vi "Relay Command Generator.vi"(1 "Relay":u16(ring) items=["1", "2", "3", "4", "5", "6", "7", "8", "9", "10", "11", "12", "13", "14", "15", "16"], 3 "On/Off":bool=TRUE) -> (8 "Generated Command":string)   [LabVIEW 2018]
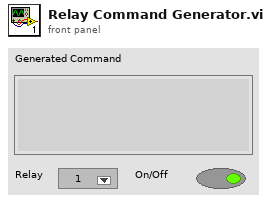
[diagram p1: front panel]
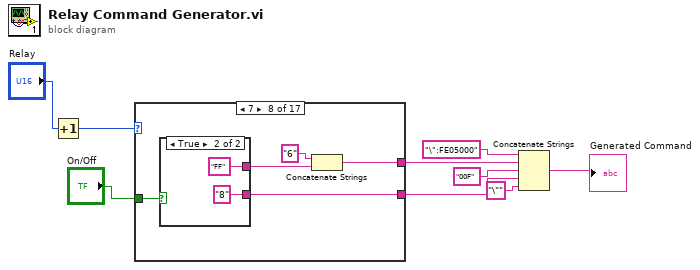
[diagram p0: block diagram]
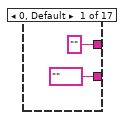
[diagram p2: hidden frame]
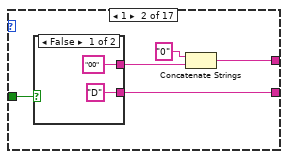
[diagram p3: hidden frame]
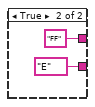
[diagram p4: hidden frame]
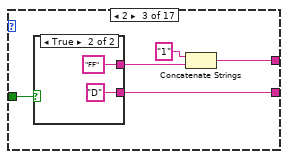
[diagram p5: hidden frame]
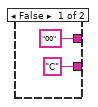
[diagram p6: hidden frame]
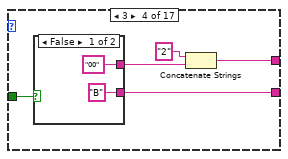
[diagram p7: hidden frame]
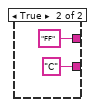
[diagram p8: hidden frame]
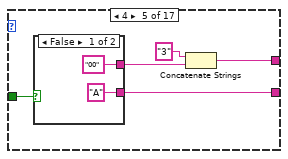
[diagram p9: hidden frame]
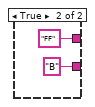
[diagram p10: hidden frame]
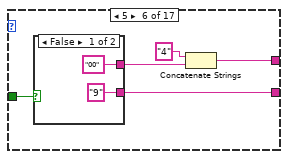
[diagram p11: hidden frame]
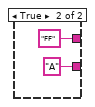
[diagram p12: hidden frame]
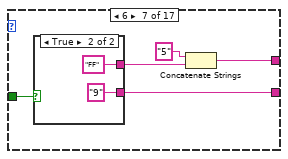
[diagram p13: hidden frame]
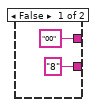
[diagram p14: hidden frame]
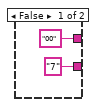
[diagram p15: hidden frame]
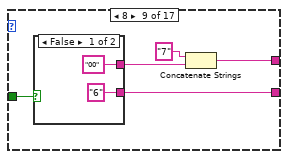
[diagram p16: hidden frame]
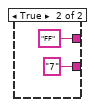
[diagram p17: hidden frame]
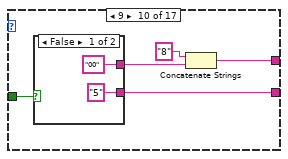
[diagram p18: hidden frame]
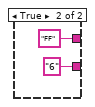
[diagram p19: hidden frame]
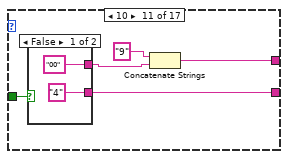
[diagram p20: hidden frame]
diagram:
  n1 = Increment(x="Relay") -> (x+1=w6:u16)
  n2 = case shown="7" w6 {
    tunnel: ["" w12 w21 w30 w39 w48 w57 w66 w75 w84 w93 w102 w111 w120 w129 w138 w147] -> w4
    tunnel: ["" w16 w25 w34 w43 w52 w61 w70 w79 w88 w97 w106 w115 w124 w133 w142 w151] -> w5
    tunnel: "On/Off" -> [_ w15 w24 w33 w42 w51 w60 w69 w78 w87 w96 w105 w114 w123 w132 w141 w150]
    frame 0, Default {
    }
    frame 1 {
      n3 = case shown="False" w15 {
        tunnel: ["00" "FF"] -> w13
        tunnel: ["D" "E"] -> w16
        frame False {
        }
        frame True {
        }
      }
      n4 = Concatenate Strings("0", w13) -> (w12:string)
    }
    frame 2 {
      n5 = case shown="True" w24 {
        tunnel: ["00" "FF"] -> w22
        tunnel: ["C" "D"] -> w25
        frame False {
        }
        frame True {
        }
      }
      n6 = Concatenate Strings("1", w22) -> (w21:string)
    }
    frame 3 {
      n7 = case shown="False" w33 {
        tunnel: ["00" "FF"] -> w31
        tunnel: ["B" "C"] -> w34
        frame False {
        }
        frame True {
        }
      }
      n8 = Concatenate Strings("2", w31) -> (w30:string)
    }
    frame 4 {
      n9 = case shown="False" w42 {
        tunnel: ["00" "FF"] -> w40
        tunnel: ["A" "B"] -> w43
        frame False {
        }
        frame True {
        }
      }
      n10 = Concatenate Strings("3", w40) -> (w39:string)
    }
    frame 5 {
      n11 = case shown="False" w51 {
        tunnel: ["00" "FF"] -> w49
        tunnel: ["9" "A"] -> w52
        frame False {
        }
        frame True {
        }
      }
      n12 = Concatenate Strings("4", w49) -> (w48:string)
    }
    frame 6 {
      n13 = case shown="True" w60 {
        tunnel: ["00" "FF"] -> w58
        tunnel: ["8" "9"] -> w61
        frame False {
        }
        frame True {
        }
      }
      n14 = Concatenate Strings("5", w58) -> (w57:string)
    }
    frame 7 {
      n15 = case shown="True" w69 {
        tunnel: ["00" "FF"] -> w67
        tunnel: ["7" "8"] -> w70
        frame False {
        }
        frame True {
        }
      }
      n16 = Concatenate Strings("6", w67) -> (w66:string)
    }
    frame 8 {
      n17 = case shown="False" w78 {
        tunnel: ["00" "FF"] -> w76
        tunnel: ["6" "7"] -> w79
        frame False {
        }
        frame True {
        }
      }
      n18 = Concatenate Strings("7", w76) -> (w75:string)
    }
    frame 9 {
      n19 = case shown="False" w87 {
        tunnel: ["00" "FF"] -> w85
        tunnel: ["5" "6"] -> w88
        frame False {
        }
        frame True {
        }
      }
      n20 = Concatenate Strings("8", w85) -> (w84:string)
    }
    frame 10 {
      n21 = case shown="False" w96 {
        tunnel: ["00" "FF"] -> w94
        tunnel: ["4" "5"] -> w97
        frame False {
        }
        frame True {
        }
      }
      n22 = Concatenate Strings("9", w94) -> (w93:string)
    }
    frame 11 {
      n23 = case shown="False" w105 {
        tunnel: ["00" "FF"] -> w103
        tunnel: ["3" "4"] -> w106
        frame False {
        }
        frame True {
        }
      }
      n24 = Concatenate Strings("A", w103) -> (w102:string)
    }
    frame 12 {
      n25 = case shown="True" w114 {
        tunnel: ["00" "FF"] -> w112
        tunnel: ["2" "3"] -> w115
        frame False {
        }
        frame True {
        }
      }
      n26 = Concatenate Strings("B", w112) -> (w111:string)
    }
    frame 13 {
      n27 = case shown="False" w123 {
        tunnel: ["00" "FF"] -> w121
        tunnel: ["1" "2"] -> w124
        frame False {
        }
        frame True {
        }
      }
      n28 = Concatenate Strings("C", w121) -> (w120:string)
    }
    frame 14 {
      n29 = case shown="False" w132 {
        tunnel: ["00" "FF"] -> w130
        tunnel: ["0" "1"] -> w133
        frame False {
        }
        frame True {
        }
      }
      n30 = Concatenate Strings("D", w130) -> (w129:string)
    }
    frame 15 {
      n31 = case shown="True" w141 {
        tunnel: ["00" "FF"] -> w139
        tunnel: ["F" "0"] -> w142
        frame False {
        }
        frame True {
        }
      }
      n32 = Concatenate Strings("E", w139) -> (w138:string)
    }
    frame 16 {
      n33 = case shown="False" w150 {
        tunnel: ["00" "FF"] -> w148
        tunnel: ["E" "F"] -> w151
        frame False {
        }
        frame True {
        }
      }
      n34 = Concatenate Strings("F", w148) -> (w147:string)
    }
  }
  n35 = Concatenate Strings("\":FE05000", w4, "00F", w5, "\"") -> (→"Generated Command":string)
